vi "initialize.vi"(8 "error in (no error)":errorcluster caption="错误输入（无错误）", 11 "6510 输入":refnum<class "6510.lvclass">) -> (0 "error out":errorcluster caption="错误输出", 3 "6510 输出":refnum<class "6510.lvclass">)   [LabVIEW 2021, in "6510.lvclass"]
uses:
  6510.lvclass
  6510.lvclass/6510.ctl
  <instrlib>/Keithley DMM6500 DAQ6500 Series/Keithley DMM6500 DAQ6500 Series.lvlib
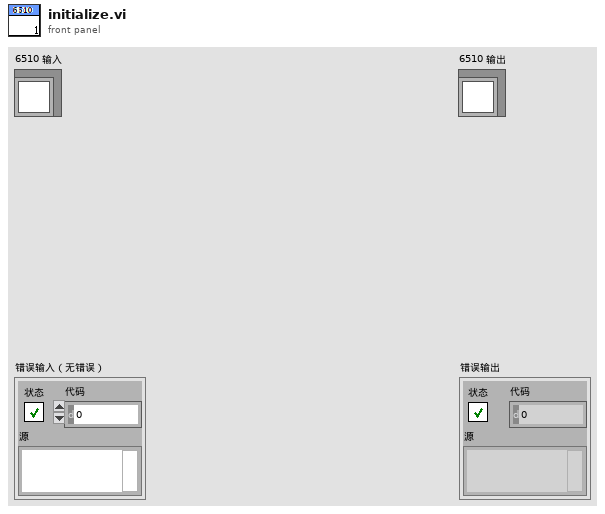
[diagram p1: front panel]
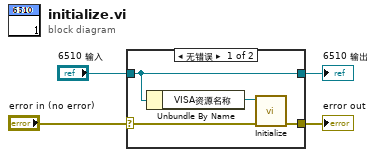
[diagram p0: block diagram]
diagram:
  n1 = case shown="无错误" "error in (no error)" {
    selector: "error in (no error)" -> [w6 w9]
    tunnel: "6510 输入" -> [w7 w10]
    tunnel: [w7 w10] -> w2
    tunnel: [w5 w9] -> w1
    frame No Error {
      n2 = Unbundle By Name(w7) -> ("VISA资源名称"=w8:refnum<visa-resource-name>)
      n3 = call <instrlib>:"Initialize.vi"("error in (no error)"=w6, "VISA resource name"=w8) -> ("error out"=w5:errorcluster)  [unwired: 8 in, 1 out]
    }
    frame Error {
    }
  }
  "error out" <- w1
  "6510 输出" <- w2
